vi "MenuSelection Response.vi"(6 "Coords":T1, 8 "error in (no error)":errorcluster, 9 "Menu Name":string, 10 "Menu Tag":string, 11 "Editor Handler in":refnum<class "Image Editor Handler.lvclass">) -> (0 "error out":errorcluster, 3 "Editor Handler out":refnum<class "Image Editor Handler.lvclass">)   [LabVIEW 2015, in "LV Image Editor Framework.lvlib" / "Image Editor Handler.lvclass"]
uses:
  Image Editor Handler.lvclass
  <vilib>/Utility/miscctls.llb/LVPoint32TypeDef.ctl
  Forms/Selection/Selection.lvclass
  Image Editor Handler.lvclass/Image Editor Handler.ctl
  Forms/Selection/Selection.lvclass/Selection.ctl
  Forms/Selection/Read Selected Shape.vi
  Forms/Shape/Shape.lvclass
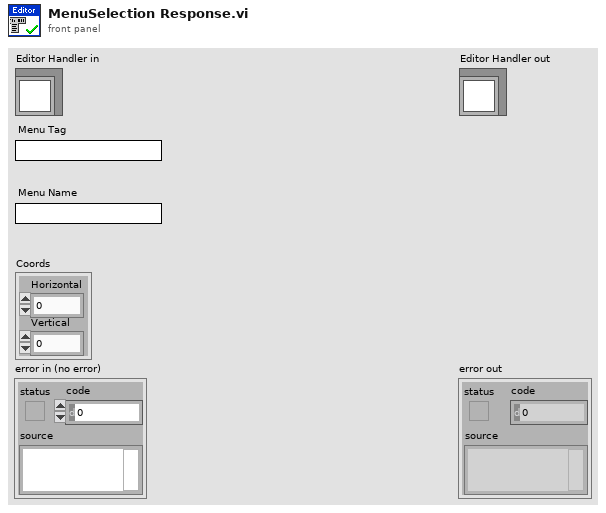
[diagram p1: front panel]
types:
  T1 = typedef "LVPoint32TypeDef.ctl" = cluster{"Horizontal":i32, "Vertical":i32}
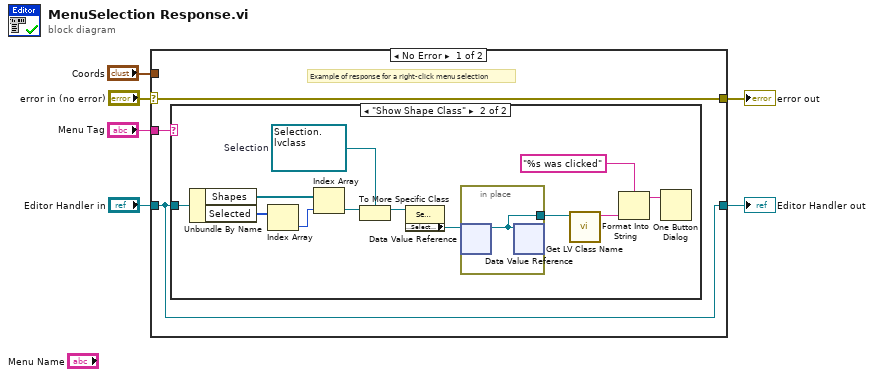
[diagram p0: block diagram]
diagram:
  n1 = case shown="No Error" "error in (no error)" {
    selector: "error in (no error)" -> [w9 w24]
    tunnel: [w9 w24] -> w5
    tunnel: [w7 w23] -> w3
    tunnel: "Editor Handler in" -> [w7 w23]
    tunnel: "Menu Tag" -> [w8 _]
    tunnel: "Coords" -> [_ _]
    frame No Error {
      # "Example of response for a right-click menu selection"
      n2 = case shown="\"Show Shape Class\"" w8 {
        tunnel: w7 -> [_ w21]
        frame Default {
        }
        frame "Show Shape Class" {
          w16 = refnum<data-value> refnum  # Selection
          n3 = Unbundle By Name(w21) -> ("Shapes"=w19:refnum<data-value>[], "Selected"=w20:i16[])
          n4 = Index Array(array=w20) -> (element=w18:i16)  [unwired: 1 in]
          n5 = Index Array(array=w19, index=w18) -> (element=w15:refnum<data-value>)
          n6 = To More Specific Class(target class=w16, reference=w15) -> (specific class reference=w14:refnum<data-value>)  [unwired: 1 in, 1 out]
          n7 = property class="Selection.lvclass"(reference=w14) -> ("Accessors:Selected Shape"=w13:refnum<data-value>)  [unwired: 1 in, 2 out]
          n8 = in-place {
            in-place-border: [w22] -> w17
            n9 = in-place-dvr #1(w13) -> (w22:refnum<class "Shape.lvclass">)  [unwired: 1 out]
            n10 = in-place-dvr #1(w22) -> ()  [unwired: 2 out]
          }
          n11 = call <vilib>:"Get LV Class Name.vi"("object"=w17) -> ("class name"=w10:string)  [unwired: 9 in, 1 out]
          n12 = Format Into String(format string="%s was clicked", w10) -> (resulting string=w12:string)  [unwired: 2 in, 1 out]
          n13 = One Button Dialog(message=w12) -> ()  [unwired: 1 in, 1 out]
        }
      }
    }
    frame Error {
    }
  }
  "error out" <- w5
  "Editor Handler out" <- w3
